vi "DBL High Pass.vi"(7 "Threshold":dbl format="%#_f", 11 "DBL In":dbl[](array[numeric]) format="%#_f") -> (3 "DBL Out":dbl[](array[numeric]) format="%#_f")   [LabVIEW 2024]
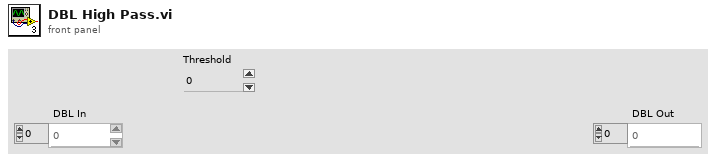
[diagram p1: front panel]
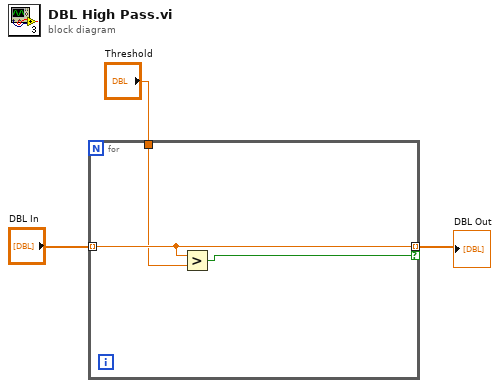
[diagram p0: block diagram]
diagram:
  n1 = for {
    tunnel: "DBL In" -> [w6] mode=indexing
    tunnel: [w6] -> w2 mode=indexing if=w4
    tunnel: "Threshold" -> [w5]
    n2 = Greater?(x=w6, y=w5) -> (0:w4:bool)
  }
  "DBL Out" <- w2
